vi "Read Analogue.vi"(8 "error in (no error)":errorcluster, 11 "Keysight 5700C in":refnum<class "Keysight 5700C.lvclass">) -> (0 "error out":errorcluster, 2 "Measurements":dbl, 3 "Keysight 5700C out":refnum<class "Keysight 5700C.lvclass">)   [LabVIEW 2021, in "Concrete.lvlib" / "Keysight 5700C.lvclass"]
uses:
  Keysight 5700C.lvclass
  Keysight 5700C.lvclass/Keysight 5700C.ctl
  Harware Abstraction/AnalogIO/AIO.lvclass
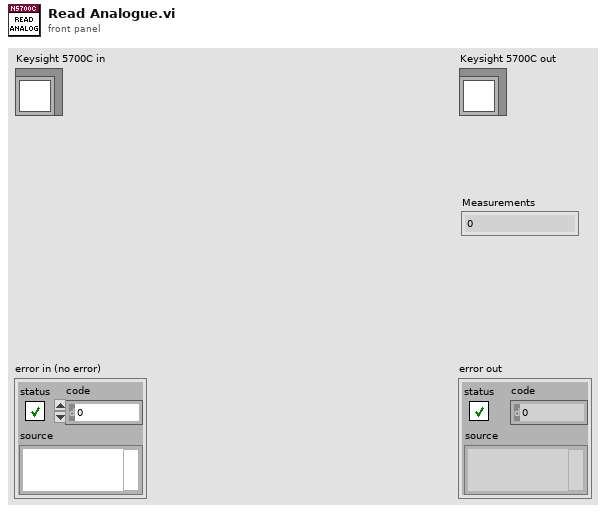
[diagram p1: front panel]
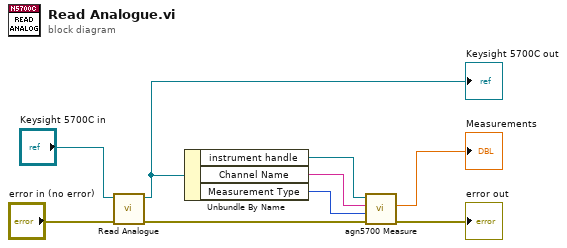
[diagram p0: block diagram]
diagram:
  n1 = call-parent "Read Analogue.vi"("error in (no error)"="error in (no error)", "PS in"="Keysight 5700C in") -> ("error out"=w3:errorcluster, "PS out"=w7:refnum<class "Keysight 5700C.lvclass">)  [unwired: 7 in, 1 out]
  "Keysight 5700C out" <- w7
  n2 = Unbundle By Name(w7) -> ("instrument handle"=w4:refnum<k15>, "Channel Name"=w5:string, "Measurement Type"=w6:i32)
  n3 = call <instrlib>:"agn5700 Measure.vi"("error in (no error)"=w3, "measurement type (Voltage)"=w6, "channel name (\"\")"=w5, "instrument handle"=w4) -> ("error out"=→"error out":errorcluster, "measurement"=→"Measurements":dbl)  [unwired: 6 out]
